vi "Controller Generate Addresses Filter Coefficients.vi"(8 "error in (no error)":errorcluster, 10 "Base address":u16=10, 11 "Coefficients":fxp<+/-,20,2>[](array[numeric])) -> (0 "error out":errorcluster, 1 "Data":fxp<+/-,20,2>, 2 "Address":u16, 3 "All coefficients loaded?":bool)   [LabVIEW 2011, in "Controller VIs.lvlib"]
uses:
  Controller VIs.lvlib
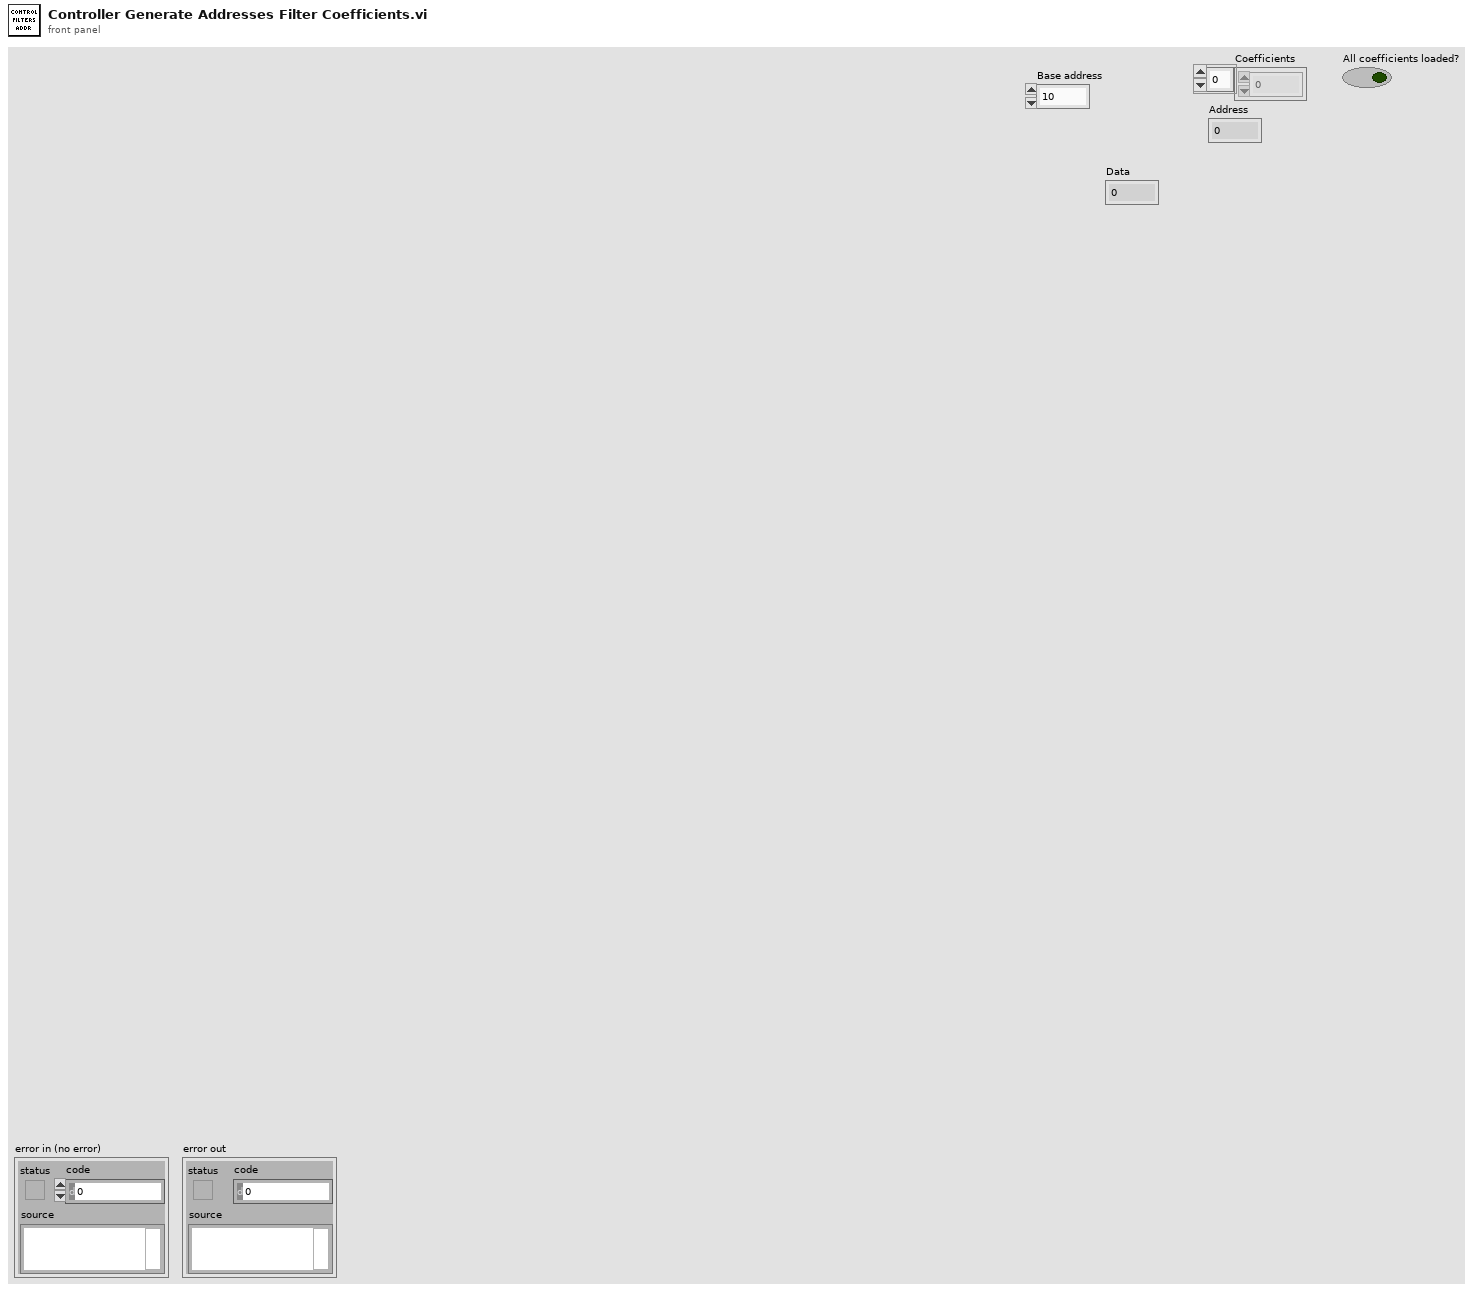
[diagram p1: front panel]
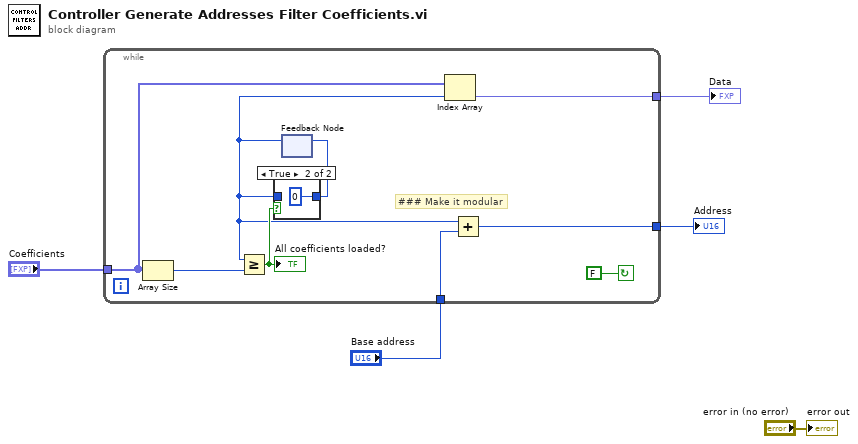
[diagram p0: block diagram]
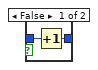
[diagram p2: hidden frame]
diagram:
  n1 = while {
    tunnel: "Coefficients" -> [w9]
    tunnel: [w11] -> w3
    tunnel: [w10] -> w2
    tunnel: "Base address" -> [w6]
    stop <- FALSE continue-if-true
    # "### Make it modular"
    n2 = Array Size(array=w9) -> (size(s)=w8:i32)
    n3 = feedback #1() -> (w7:u16)  [unwired: 1 in]
    n4 = Greater Or Equal?(x=w7, y=w8) -> (x >= y?=w14:bool)
    "All coefficients loaded?" <- w14
    n5 = case shown="True" w14 {
      tunnel: w7 -> [w16 _]
      tunnel: [w15 u16 0] -> w13
      frame False {
        n6 = Increment(x=w16) -> (x+1=w15:u16)
      }
      frame True {
      }
    }
    n7 = feedback-in #1(w13) -> ()
    n8 = Index Array(array=w9, index=w7) -> (element=w10:fxp<+/-,20,2>)
    n9 = Add(x=w7, y=w6) -> (x+y=w11:u16)
  }
  "Address" <- w3
  "Data" <- w2
  "error out" <- "error in (no error)"
